vi "2D tilted Gaussian model.vi"(3 "output control":T1, 4 "data":variant, 5 "X":dbl[](array[numeric]), 6 "a":dbl[](array[numeric])) -> (0 "error out":errorcluster, 1 "f'(X,a)":dbl[][](array[numeric]), 2 "f(X,a)":dbl[](array[numeric]))   [LabVIEW 2024]
doc: "Gaussian surface with offset model"
uses:
  <vilib>/gmath/NumericalOptimization/LM_output select.ctl
  <vilib>/gmath/NI_Gmath.lvlib
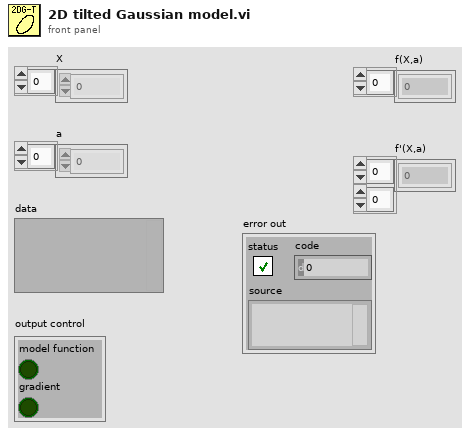
[diagram p1: front panel]
types:
  T1 = typedef "NI_Gmath.lvlib/LM_output select.ctl" = cluster{"model function":bool, "gradient":bool}
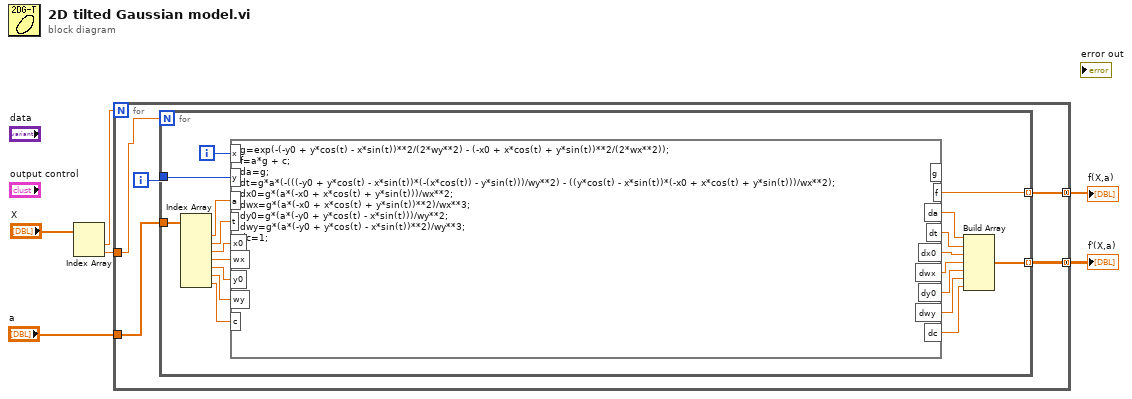
[diagram p0: block diagram]
diagram:
  n1 = Index Array(array="X") -> (element #1=w2:dbl, element #2=w1:dbl)  [unwired: 2 in]
  n2 = for {
    N: w2 -> [_]
    tunnel: "a" -> [w11]
    tunnel: [w10] -> w5 mode=concatenating
    tunnel: [w9] -> w4 mode=concatenating
    tunnel: w1 -> [w7]
    i -> [w8]
    n3 = for {
      N: w7 -> [_]
      tunnel: w11 -> [w23]
      tunnel: [w15] -> w10 mode=indexing
      tunnel: [w14] -> w9 mode=indexing
      tunnel: w8 -> [w12]
      i -> [w13]
      n4 = Index Array(array=w23) -> (element #1=w24:dbl, element #2=w25:dbl, element #3=w26:dbl, element #4=w27:dbl, element #5=w28:dbl, element #6=w29:dbl, element #7=w30:dbl)  [unwired: 7 in]
      n5 = formula code="g=exp(-(-y0 + y*cos(t) - x*sin(t))**2/(2*wy**2) - (-x0 + x*cos(t) + y*sin(t))**2/(2*wx**2));\nf=a*g + c;\nda=g;\ndt=g*a*(-(((-y0 + y*cos(t) - x*sin(t))*(-(x*cos(t)) - y*sin(t)))/wy**2) - ((y*cos(t) - x*sin(t))*(-x0 + x*cos(t) + y*sin(t)))/wx**2);\ndx0=g*(a*(-x0 + x*cos(t) + y*sin(t)))/wx**2;\ndwx=g*(a*(-x0 + x*cos(t) + y*sin(t))**2)/wx**3;\ndy0=g*(a*(-y0 + y*cos(t) - x*sin(t)))/wy**2;\ndwy=g*(a*(-y0 + y*cos(t) - x*sin(t))**2)/wy**3;\ndc=1;"("x"=w13, "a"=w24, "t"=w25, "x0"=w26, "wx"=w27, "y0"=w28, "wy"=w29, "c"=w30, "y"=w12) -> ("f"=w15:dbl, "da"=w22:dbl, "dt"=w21:dbl, "dx0"=w20:dbl, "dwx"=w19:dbl, "dy0"=w18:dbl, "dwy"=w17:dbl, "dc"=w16:dbl)  [unwired: 1 out]
      n6 = Build Array(w22, w21, w20, w19, w18, w17, w16) -> (w14:dbl[])
    }
  }
  "f(X,a)" <- w5
  "f'(X,a)" <- w4
